vi "runScript.vi"(6 "timeStamp":string, 8 "error in (no error)":errorcluster, 9 "Path":path, 10 "CompiledScript":T1, 11 "AtomChipHWC in":refnum<class "AtomChipHWC.lvclass">) -> (0 "error out":errorcluster, 3 "AtomChipHWC out":refnum<class "AtomChipHWC.lvclass">)   [LabVIEW 2009, in "Hardware.lvlib" / "HWControllers.lvlib" / "AtomChipHWC.lvclass"]
uses:
  AtomChipHWC.lvclass
  Tools/SettingsProcessors/ScriptListCompiler/ScriptListCompiler.lvclass
  Channels/VoltOutput/AnalogOutput.lvclass
  Channels/Digital/DigitalOutput.lvclass
  Channels/DDSOutput/Generic/DDSOutput.lvclass
  AtomChipHWC.lvclass/AtomChipHWC.ctl
  HWController.lvclass
  HardwareConfiguration/HWConfiguration.lvclass
panel:
  out "Analog time":dbl
  out "DDS time":dbl
  out "Digital Time":dbl
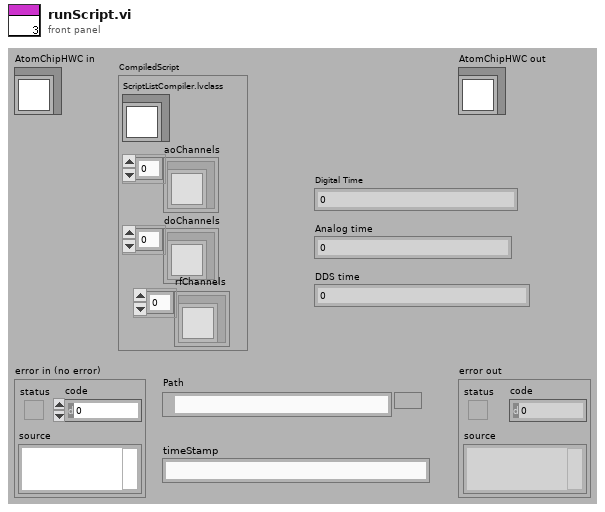
[diagram p1: front panel]
types:
  T1 = cluster{"ScriptListCompiler.lvclass":refnum<class "ScriptListCompiler.lvclass">, "aoChannels":refnum<class "AnalogOutput.lvclass">[], "doChannels":refnum<class "DigitalOutput.lvclass">[], "rfChannels":refnum<class "DDSOutput.lvclass">[]}
  T2 = enum16{"Ready", "Compiling", "Configured", "Running", "Stopping", "Unresolved Error"}
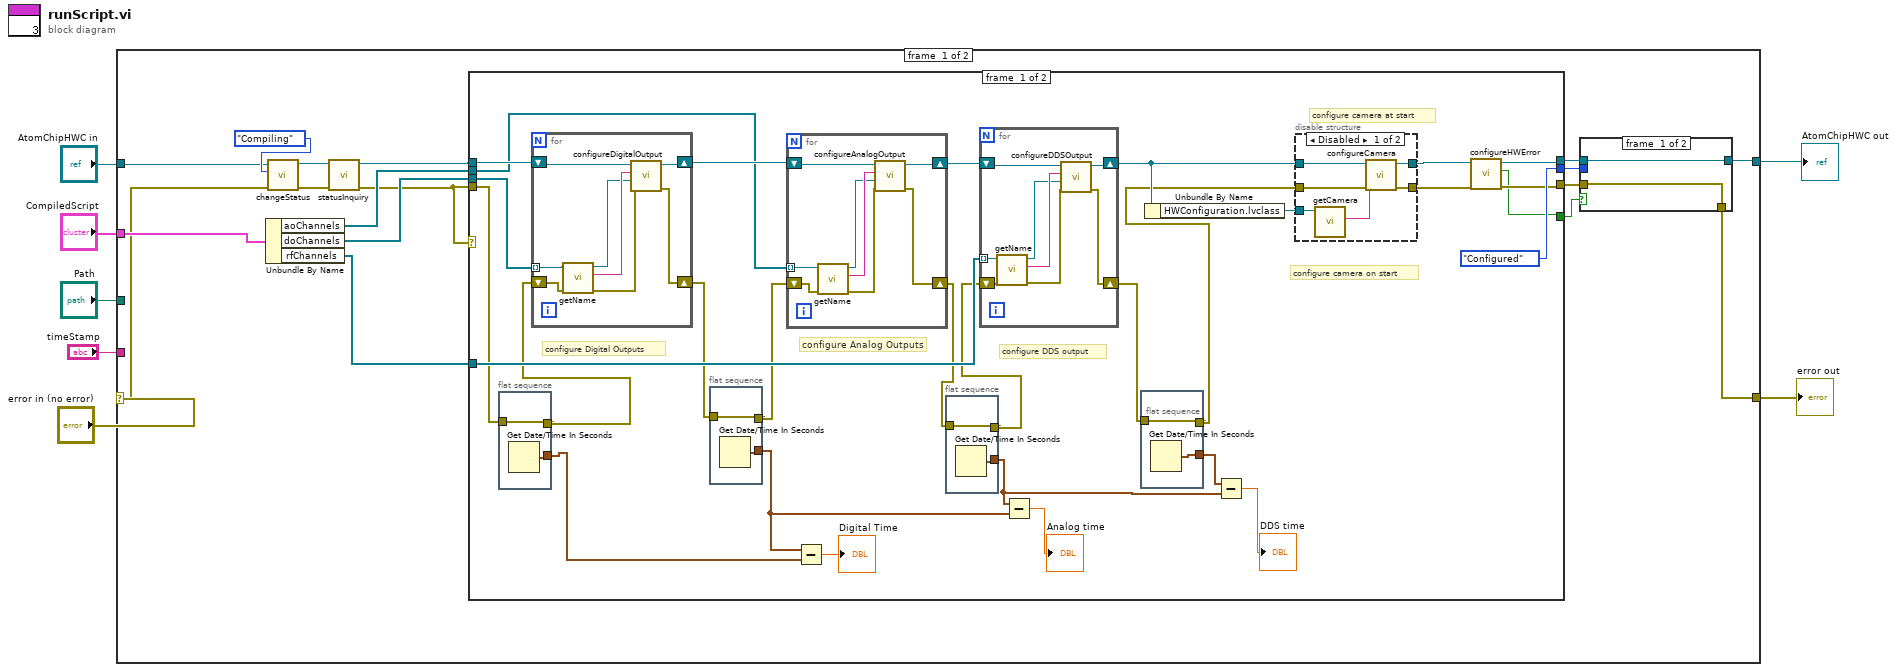
[diagram p0: block diagram]
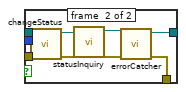
[diagram p2: hidden frame]
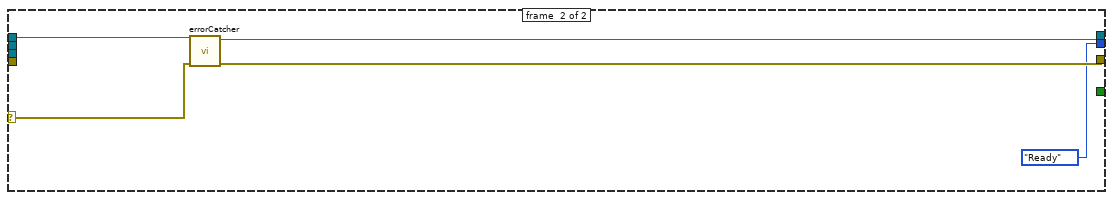
[diagram p4: hidden frame]
diagram:
  n1 = case shown="No Error" "error in (no error)" {
    selector: "error in (no error)" -> [w8 w110]
    tunnel: "AtomChipHWC in" -> [w9 w111]
    tunnel: [w13 w111] -> w5
    tunnel: [w12 w110] -> w4
    tunnel: "CompiledScript" -> [w18 _]
    tunnel: "timeStamp" -> [_ _]
    tunnel: "Path" -> [_ _]
    frame #0 {
      n2 = Unbundle By Name(w18) -> ("aoChannels"=w16:refnum<class "AnalogOutput.lvclass">[], "doChannels"=w17:refnum<class "DigitalOutput.lvclass">[], "rfChannels"=w11:refnum<class "DDSOutput.lvclass">[])
      n3 = call "changeStatus.vi"("error in (no error)"=w8, "status"=T2."Compiling", "HWController in"=w9) -> ("error out"=w22:errorcluster, "HWController out"=w21:refnum<class "AtomChipHWC.lvclass">)  [unwired: 7 in]
      n4 = call-dynamic "statusInquiry.vi"("error in (no error)"=w22, "HWController in"=w21) -> ("error out"=w14:errorcluster, "HWController out"=w15:refnum<class "AtomChipHWC.lvclass">)  [unwired: 8 in]
      n5 = case shown="No Error" w14 {
        selector: w14 -> [_ w106]
        tunnel: [w52 w108] -> w24
        tunnel: [w53 w107] -> w23
        tunnel: w15 -> [w63 w109]
        tunnel: w14 -> [w50 _]
        tunnel: w17 -> [w62 _]
        tunnel: w16 -> [w61 _]
        tunnel: [T2."Configured" ("status") T2."Ready" ("status")] -> w19
        tunnel: w11 -> [w59 _]
        tunnel: [w51 _] -> w10
        frame #0 {
          # "configure DDS output"
          # "configure camera at start"
          # "configure camera on start"
          # "configure Analog Outputs"
          # "configure Digital Outputs"
          n6 = flat-sequence {
            tunnel: [w72] -> w49
            tunnel: w50 -> [w72]
            tunnel: [w71] -> w44
            frame #0 {
              n7 = Get Date/Time In Seconds() -> (seconds since 1Jan1904=w71:timestamp)
            }
          }
          n8 = for {
            shift-right: [w98] -> w48
            shift-left: w49 -> [w104]
            shift-right: [w102] -> w64
            shift-left: w63 -> [w103]
            tunnel: w62 -> [w97] mode=indexing
            n9 = call-dynamic "getName.vi"("error in (no error)"=w104, "DigitalOutput.lvclass in"=w97) -> ("error out"=w100:errorcluster, "name"=w101:string, "DigitalOutput.lvclass out"=w99:refnum<class "DigitalOutput.lvclass">)  [unwired: 7 in]
            n10 = call "configureDigitalOutput.vi"("error in (no error)"=w100, "DigitalOutput"=w99, "deviceName"=w101, "AtomChipHWC in"=w103) -> ("error out"=w98:errorcluster, "AtomChipHWC out"=w102:refnum<class "AtomChipHWC.lvclass">)  [unwired: 6 in]
          }
          n11 = flat-sequence {
            tunnel: [w70] -> w47
            tunnel: w48 -> [w70]
            tunnel: [w69] -> w42
            frame #0 {
              n12 = Get Date/Time In Seconds() -> (seconds since 1Jan1904=w69:timestamp)
            }
          }
          n13 = for {
            tunnel: w61 -> [w89] mode=indexing
            shift-right: [w93] -> w46
            shift-left: w47 -> [w96]
            shift-right: [w94] -> w58
            shift-left: w64 -> [w95]
            n14 = call "getName.vi"("error in (no error)"=w96, "AnalogOutput.lvclass in"=w89) -> ("error out"=w92:errorcluster, "name"=w91:string, "AnalogOutput.lvclass out"=w90:refnum<class "AnalogOutput.lvclass">)  [unwired: 7 in]
            n15 = call "configureAnalogOutput.vi"("error in (no error)"=w92, "AnalogOutput"=w90, "deviceName"=w91, "AtomChipHWC in"=w95) -> ("error out"=w93:errorcluster, "AtomChipHWC out"=w94:refnum<class "AtomChipHWC.lvclass">)  [unwired: 6 in]
          }
          n16 = Subtract(x=w42, y=w44) -> (x-y=→"Digital Time":dbl)
          n17 = flat-sequence {
            tunnel: [w68] -> w45
            tunnel: w46 -> [w68]
            tunnel: [w67] -> w38
            frame #0 {
              n18 = Get Date/Time In Seconds() -> (seconds since 1Jan1904=w67:timestamp)
            }
          }
          n19 = for {
            tunnel: w59 -> [w88] mode=indexing
            shift-right: [w83] -> w41
            shift-left: w45 -> [w87]
            shift-right: [w85] -> w57
            shift-left: w58 -> [w86]
            n20 = call-dynamic "getName.vi"("error in (no error)"=w87, "DDSOutput in"=w88) -> ("error out"=w84:errorcluster, "name"=w82:string, "DDSOutput out"=w81:refnum<class "DDSOutput.lvclass">)  [unwired: 7 in]
            n21 = call "configureDDSOutput.vi"("error in (no error)"=w84, "DDSOutput"=w81, "device"=w82, "AtomChipHWC in"=w86) -> ("error out"=w83:errorcluster, "AtomChipHWC out"=w85:refnum<class "AtomChipHWC.lvclass">)  [unwired: 6 in]
          }
          n22 = Subtract(x=w38, y=w42) -> (x-y=→"Analog time":dbl)
          n23 = flat-sequence {
            tunnel: [w66] -> w40
            tunnel: w41 -> [w66]
            tunnel: [w65] -> w39
            frame #0 {
              n24 = Get Date/Time In Seconds() -> (seconds since 1Jan1904=w65:timestamp)
            }
          }
          n25 = Unbundle By Name(w57) -> ("HWConfiguration.lvclass"=w56:refnum<class "HWConfiguration.lvclass">)
          n26 = Subtract(x=w39, y=w38) -> (x-y=→"DDS time":dbl)
          n27 = disable-structure shown="Disabled" {
            disable-tunnel: w40 -> [w78 w79]
            disable-tunnel: [w77 w80] -> w55
            disable-tunnel: [w76 w79] -> w54
            disable-tunnel: w57 -> [w75 w80]
            disable-tunnel: w56 -> [w74 _]
            frame #0 {
              n28 = call-dynamic "getCamera.vi"("HWConfiguration.lvclass in"=w74) -> ("camera"=w73:string)  [unwired: 8 in, 2 out]
              n29 = call "configureCamera.vi"("error in (no error)"=w78, "device"=w73, "AtomChipHWC in"=w75) -> ("error out"=w76:errorcluster, "AtomChipHWC out"=w77:refnum<class "AtomChipHWC.lvclass">)  [unwired: 7 in]
            }
            frame #1 {
            }
          }
          n30 = call-dynamic "configureHWError.vi"("error in (no error)"=w54, "AtomChipHWC in"=w55) -> ("error out"=w53:errorcluster, "error"=w51:bool, "AtomChipHWC out"=w52:refnum<class "AtomChipHWC.lvclass">)  [unwired: 7 in]
        }
        frame #1 {
          n31 = call-dynamic "errorCatcher.vi"("error in (no error)"=w106, "HWController in"=w109) -> ("error out"=w107:errorcluster, "HWController out"=w108:refnum<class "AtomChipHWC.lvclass">)  [unwired: 8 in]
        }
      }
      n32 = case shown="False" w10 {
        tunnel: w24 -> [w26 w35]
        tunnel: w23 -> [w25 w34]
        tunnel: w19 -> [_ w31]
        tunnel: [w26 w28] -> w13
        tunnel: [w25 w27] -> w12
        frame #0 {
        }
        frame #1 {
          n33 = call "changeStatus.vi"("error in (no error)"=w34, "status"=w31, "HWController in"=w35) -> ("error out"=w33:errorcluster, "HWController out"=w32:refnum<class "AtomChipHWC.lvclass">)  [unwired: 7 in]
          n34 = call-dynamic "statusInquiry.vi"("error in (no error)"=w33, "HWController in"=w32) -> ("error out"=w29:errorcluster, "HWController out"=w30:refnum<class "AtomChipHWC.lvclass">)  [unwired: 8 in]
          n35 = call-dynamic "errorCatcher.vi"("error in (no error)"=w29, "HWController in"=w30) -> ("error out"=w27:errorcluster, "HWController out"=w28:refnum<class "AtomChipHWC.lvclass">)  [unwired: 8 in]
        }
      }
    }
    frame #1 {
    }
  }
  "error out" <- w4
  "AtomChipHWC out" <- w5
